vi "Get Display String.vi"(11 "Boolean in":refnum<class "Boolean.lvclass">) -> (2 "Display String":string)   [LabVIEW 2018, in "Boolean.lvclass"]
uses:
  Boolean.lvclass
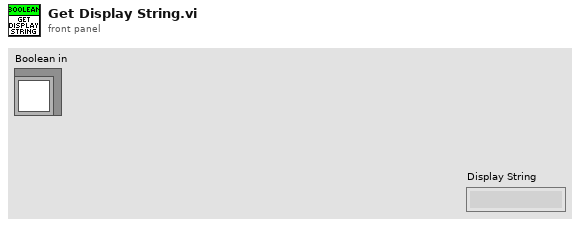
[diagram p1: front panel]
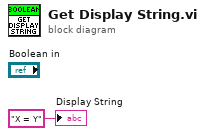
[diagram p0: block diagram]
diagram:
  "Display String" <- "X = Y" ("Display String")
